vi "ImagearrayRandom.vi"(10 "2D picture array":picture[][](array[picture])) -> (1 "mark blank":i32[](array[numeric]), 2 "random 2d picture array":picture[][](array[picture]))   [LabVIEW 2014]
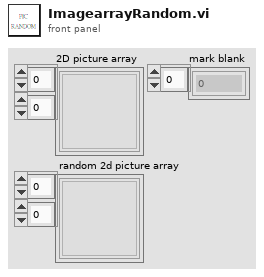
[diagram p1: front panel]
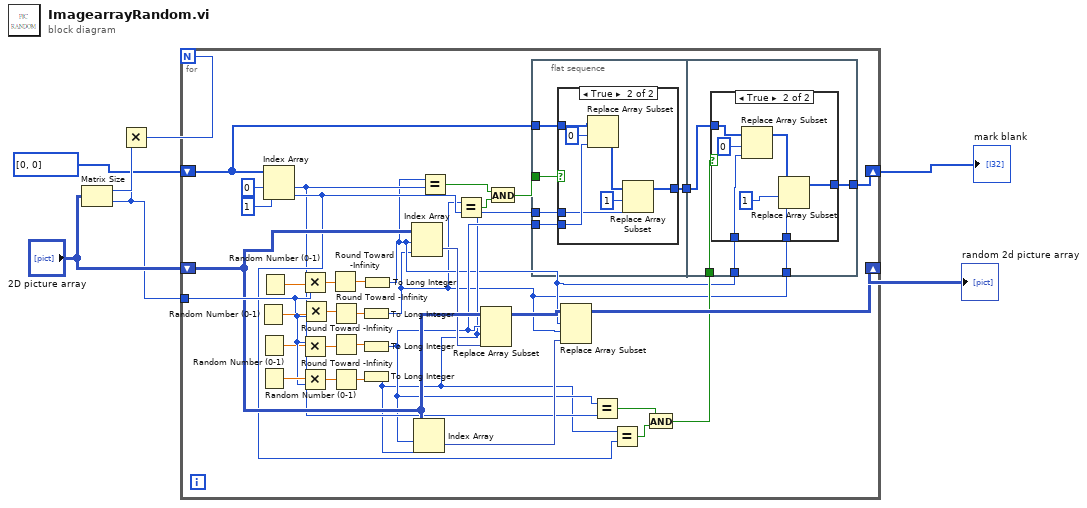
[diagram p0: block diagram]
diagram:
  n1 = Matrix Size(0:"2D picture array") -> (1:w6:i32, 2:w4:i32)
  n2 = Multiply(x=w6, y=w4) -> (x*y=w7:i32)
  n3 = for {
    N: w7 -> [_]
    shift-right: [w27] -> w3
    shift-left: "2D picture array" -> [w29]
    tunnel: w4 -> [w39]
    shift-right: [w17] -> w1
    shift-left: i32[] [0, 0] -> [w19]
    n4 = Random Number (0-1)() -> (number: 0 to 1=w40:dbl)
    n5 = Random Number (0-1)() -> (number: 0 to 1=w38:dbl)
    n6 = Random Number (0-1)() -> (number: 0 to 1=w42:dbl)
    n7 = Random Number (0-1)() -> (number: 0 to 1=w41:dbl)
    n8 = Index Array(array=w19, index #1=0 ("index"), index #2=1 ("index")) -> (element #1=w15:i32, element #2=w16:i32)
    n9 = Multiply(x=w41, y=w39) -> (x*y=w37:dbl)
    n10 = Multiply(x=w39, y=w38) -> (x*y=w35:dbl)
    n11 = Multiply(x=w42, y=w39) -> (x*y=w34:dbl)
    n12 = Multiply(x=w40, y=w39) -> (x*y=w36:dbl)
    n13 = Round Toward -Infinity(1:w37) -> (0:w33:dbl)
    n14 = Round Toward -Infinity(1:w36) -> (0:w30:dbl)
    n15 = Round Toward -Infinity(1:w35) -> (0:w32:dbl)
    n16 = Round Toward -Infinity(1:w34) -> (0:w31:dbl)
    n17 = To Long Integer(number=w30) -> (32bit integer=w8:i32)
    n18 = To Long Integer(number=w32) -> (32bit integer=w11:i32)
    n19 = To Long Integer(number=w31) -> (32bit integer=w10:i32)
    n20 = To Long Integer(number=w33) -> (32bit integer=w9:i32)
    n21 = Index Array(array=w29, index (row)=w9, index (col)=w8) -> (element=w26:picture)
    n22 = Index Array(array=w29, index (row)=w11, index (col)=w10) -> (element=w25:picture)
    n23 = Equal?(x=w9, y=w15) -> (x = y?=w21:bool)
    n24 = Equal?(x=w8, y=w16) -> (x = y?=w22:bool)
    n25 = Replace Array Subset(array=w29, new element=w26, index (row)=w11, index (col)=w10) -> (w28:picture[][])
    n26 = And(x=w21, y=w22) -> (x .and. y?=w20:bool)
    n27 = flat-sequence {
      tunnel: w20 -> [w47]
      tunnel: w19 -> [w46]
      tunnel: [w45] -> w18
      tunnel: w11 -> [w44]
      tunnel: w10 -> [w43]
      tunnel: w18 -> [w60]
      tunnel: [w59] -> w17
      tunnel: w12 -> [w58]
      tunnel: w9 -> [w57]
      tunnel: w8 -> [w56]
      frame #0 {
        n28 = case shown="True" w47 {
          tunnel: w46 -> [w48 w55]
          tunnel: [w48 w51] -> w45
          tunnel: w44 -> [_ w50]
          tunnel: w43 -> [_ w49]
          frame False {
          }
          frame True {
            n29 = Replace Array Subset(array=w55, new element=w50, index=0) -> (w54:i32[])
            n30 = Replace Array Subset(array=w54, new element=w49, index=1) -> (w51:i32[])
          }
        }
      }
      frame #1 {
        n31 = case shown="True" w58 {
          tunnel: w60 -> [w61 w68]
          tunnel: [w61 w66] -> w59
          tunnel: w57 -> [_ w63]
          tunnel: w56 -> [_ w62]
          frame False {
          }
          frame True {
            n32 = Replace Array Subset(array=w68, new element=w63, index=0) -> (w67:i32[])
            n33 = Replace Array Subset(array=w67, new element=w62, index=1) -> (w66:i32[])
          }
        }
      }
    }
    n34 = Replace Array Subset(array=w28, new element=w25, index (row)=w9, index (col)=w8) -> (w27:picture[][])
    n35 = Equal?(x=w11, y=w15) -> (x = y?=w13:bool)
    n36 = Equal?(x=w10, y=w16) -> (x = y?=w14:bool)
    n37 = And(x=w13, y=w14) -> (x .and. y?=w12:bool)
  }
  "random 2d picture array" <- w3
  "mark blank" <- w1
